vi "Get Output Channel.vi"(8 "error in (no error)":errorcluster, 11 "Output Channels[]":refnum<class "Output Channels.lvclass">[](array[class])) -> (0 "error out":errorcluster, 3 "Output Channel Details":T1={"Enable Output"=FALSE, "Channel Name"="", "Value"=1.0, "Unit"=""} {"Value" min=-422.2 max=422.2 step=1.0 format="%#.1f"})   [LabVIEW 2020, in "Plugin.lvlib" / "Plugin_UI.lvclass"]
doc: "Reads all the output channel details required for updating the Configuration Interface."
uses:
  Plugin_UI.lvclass
  Channels/Output Channels/Output Channels.lvclass
  C:/SVN_LabSys/labsys_lvcode/LabSys_SourceCode/Plugin Template/Source/Code/Channels/Plugin_Channels.lvclass
  Output Channel Config.ctl
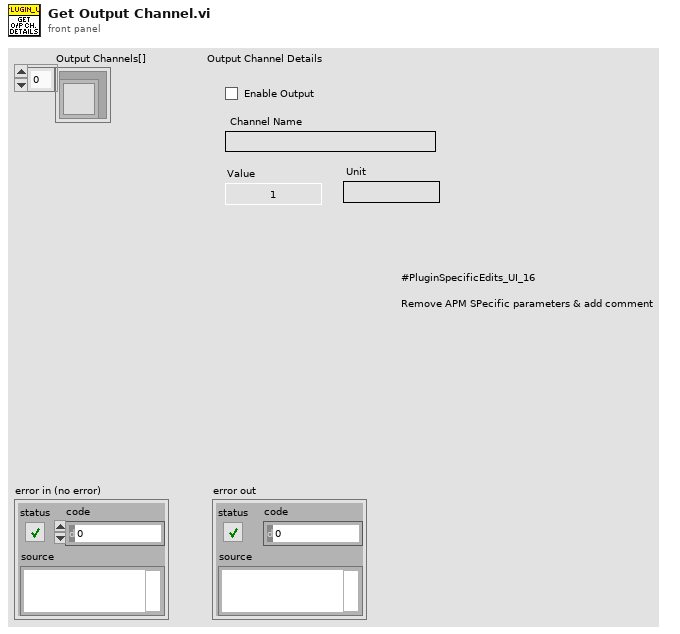
[diagram p1: front panel]
types:
  T1 = typedef "Plugin.lvlib/Plugin_UI.lvclass/Output Channel Config.ctl" = cluster{"Enable Output":bool, "Channel Name":string, "Value":dbl, "Unit":string}
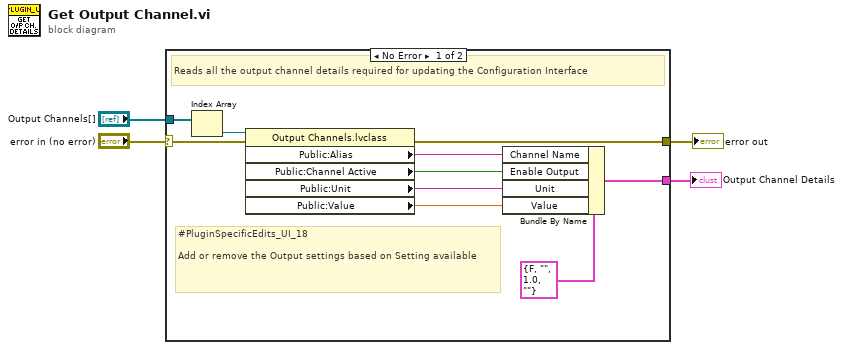
[diagram p0: block diagram]
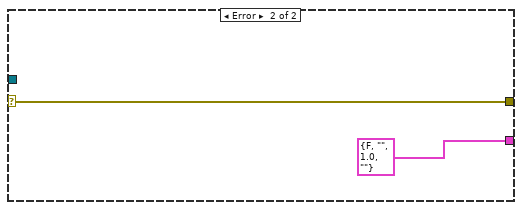
[diagram p2: hidden frame]
diagram:
  n1 = case shown="No Error" "error in (no error)" {
    selector: "error in (no error)" -> [w6 w16]
    tunnel: [w14 w16] -> w4
    tunnel: "Output Channels[]" -> [w12 _]
    tunnel: [w10 T1 {"Enable Output"=FALSE, "Channel Name"="", "Value"=1.0, "Unit"=""} ("Output Channel Details")] -> w2
    frame No Error {
      # "#PluginSpecificEdits_UI_18 \n\nAdd or remove the Output settings based on Setting available"
      # "Reads all the output channel details required for updating the Configuration Interface"
      n2 = Index Array(array=w12) -> (element=w13:refnum<class "Output Channels.lvclass">)  [unwired: 1 in]
      n3 = property class="Output Channels.lvclass"(reference=w13, error in=w6) -> (error out=w14:errorcluster, "Public:Alias"=w9:string, "Public:Channel Active"=w8:bool, "Public:Unit"=w7:string, "Public:Value"=w5:dbl)  [unwired: 1 out]
      n4 = Bundle By Name(cluster=T1 {"Enable Output"=FALSE, "Channel Name"="", "Value"=1.0, "Unit"=""} ("Output Channel Details"), "Channel Name"=w9, "Enable Output"=w8, "Unit"=w7, "Value"=w5) -> (w10:T1)
    }
    frame Error {
    }
  }
  "error out" <- w4
  "Output Channel Details" <- w2
